vi "Bounds Size Conversion.vi"(10 "Size":T2, 11 "Bounds":T1) -> (2 "Bounds Out":T1, 3 "Size Out":T2)   [LabVIEW 2011]
doc: "This VI is a simple VI that will convert from bounds, given the four points of an object, into the Width and Height, or vise versa.\n\n-------------\nDeveloped by Brian Hoover (hooovahh)"
uses:
  <vilib>/Utility/miscctls.llb/LVRectTypeDef.ctl
  <vilib>/Utility/miscctls.llb/LVBoundsTypeDef.ctl
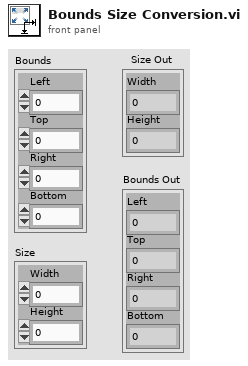
[diagram p1: front panel]
types:
  T1 = typedef "LVRectTypeDef.ctl" = cluster{"Left":i16, "Top":i16, "Right":i16, "Bottom":i16}
  T2 = typedef "LVBoundsTypeDef.ctl" = cluster{"Width":u32, "Height":u32}
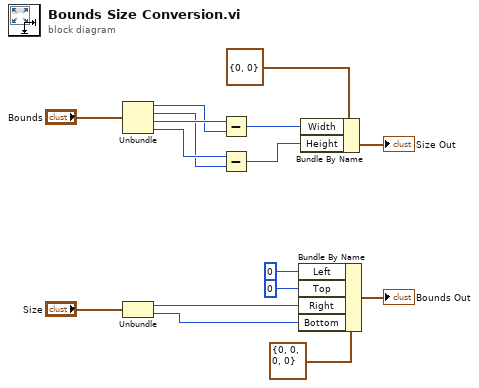
[diagram p0: block diagram]
diagram:
  n1 = Unbundle("Bounds") -> ("Left"=w13:i16, "Top"=w8:i16, "Right"=w14:i16, "Bottom"=w9:i16)
  n2 = Unbundle("Size") -> ("Width"=w2:u32, "Height"=w1:u32)
  n3 = Subtract(x=w14, y=w13) -> (x-y=w10:i16)
  n4 = Subtract(x=w9, y=w8) -> (x-y=w7:i16)
  n5 = Bundle By Name(cluster=T1 {"Left"=0, "Top"=0, "Right"=0, "Bottom"=0} ("Bounds Out"), "Left"=i16 0, "Top"=i16 0, "Right"=w2, "Bottom"=w1) -> (→"Bounds Out":T1)
  n6 = Bundle By Name(cluster=T2 {"Width"=0, "Height"=0} ("Size Out"), "Width"=w10, "Height"=w7) -> (→"Size Out":T2)
